vi "Control Documentation.vi"() -> ()   [LabVIEW 2012]
uses:
  Control Documentation.ctl
  <vilib>/regexp/Match Regular Expression.xnode
panel:
  out "error out":errorcluster
  out "Progress":i32(slide) scale=0.0..64.0
  in  "Ignore":bool
  in  "Write":bool
  in  "File Folder":path=path "C:/Users/husmith/Documents/GitHub/iWorx/LabVIEW"
  out "Found Controls":T1(array[cluster])
  in  "Control Documentation":T2[](array[typedef])=[{"Label"="Channel", "Tip Strip"="Select the iWorx sensor adaptor channel", "Description"="Select the channel for the iWorx sensor adaptor. Chanel 1 is read on AI0 channel 2 is read on AI1."}, {"Label"="Raw Signal", "Tip Strip"="The raw voltage signal from the sensor", "Description"="This control shows the raw voltage signal from the myDAQ before any scaling is applied."}, {"Label"="Sample Timing", "Tip Strip"="Select how frequently to read data", "Description"="Set the approximate read frequency for the data acquisition functions."}, {"Label"="Set Up", "Tip Strip"="Open sensor set up instructions", "Description"=""}, {"Label"="Calibration Data", "Tip Strip"="Calibration set points", "Description"="The set points are used to calulate a linear slope and offset using the formulas below.\nSlope = (X2-X1)/(Y2-Y1)\nOffset = (X1-(slope*Y1)\nScaled Data = Data*m+b"}, {"Label"="Set SP1", "Tip Strip"="Save current raw voltage as set point 1 voltage", "Description"=""}, {"Label"="Set SP2", "Tip Strip"="Save current raw voltage as set point 1 voltage", "Description"=""}, {"Label"="Slope", "Tip Strip"="The slope calculated using the calibration data", "Description"=""}, {"Label"="Offset", "Tip Strip"="The offset calculated using the calibration data", "Description"=""}, {"Label"="Autoscale Y", "Tip Strip"="Toggle Y axis autoscaling", "Description"=""}, {"Label"="Open Log", "Tip Strip"="Open the current chart data in Excel", "Description"="Note: This feature will not work if Microsoft Excel is not installed."}, {"Label"="Clear Chart", "Tip Strip"="Clear the waveform chart data", "Description"=""}, {"Label"="Processed Signal", "Tip Strip"="The scaled sensor data", "Description"=""}, {"Label"="Waveform Chart", "Tip Strip"="", "Description"=""}, {"Label"="Snapshot", "Tip Strip"="Take a snapshot of the graph and save to file", "Description"=""}, {"Label"="Pause Button", "Tip Strip"="Pause the waveform chart", "Description"=""}, {"Label"="stop", "Tip Strip"="Stop the VI", "Description"=""}]
  out "All Controls":string[](array[string])
  out "File Path Control":path=path "C:/Users/husmith/Documents/GitHub/iWorx/LabVIEW/examples/iWorx - Force.vi"
  in  "Background":bool
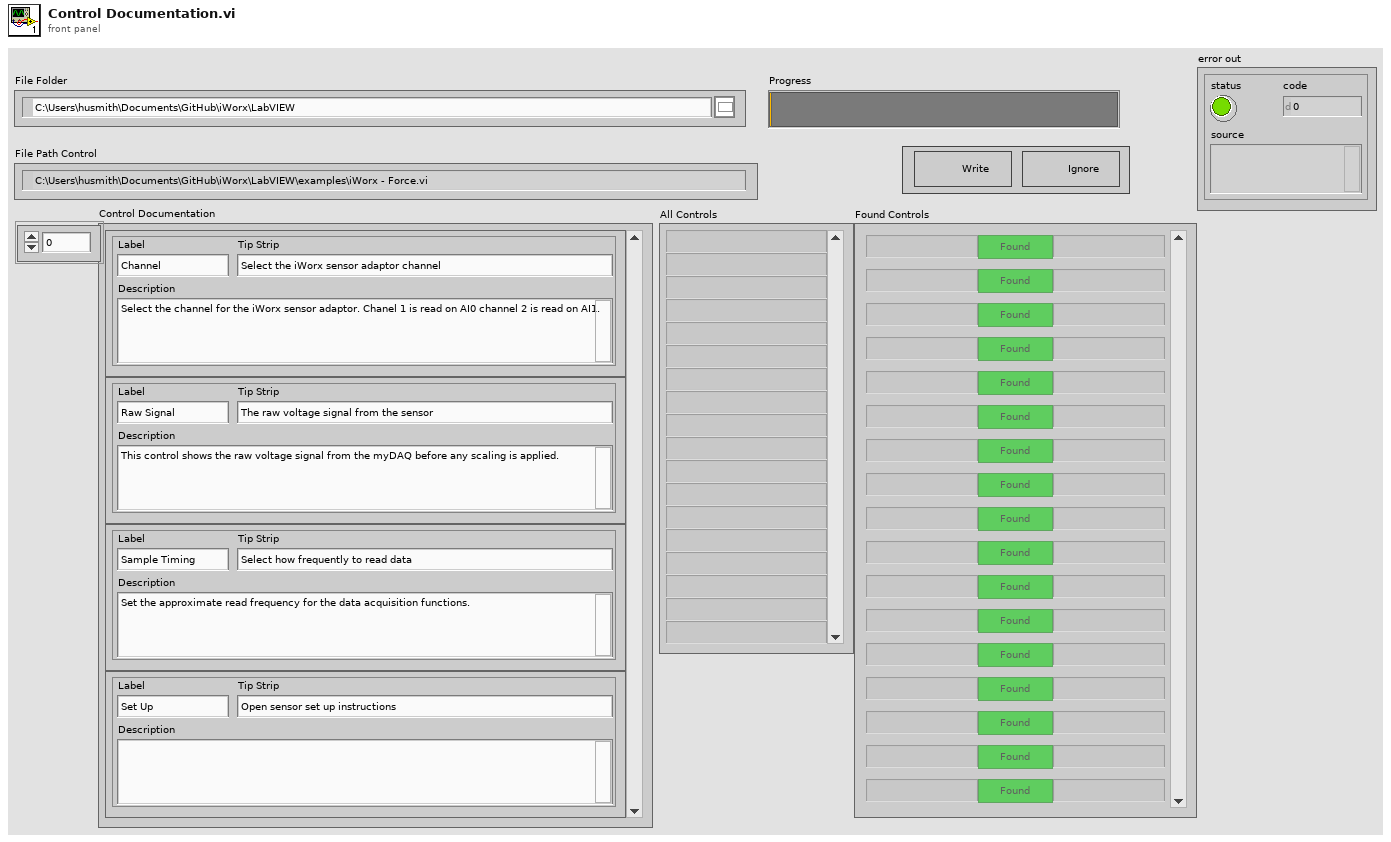
[diagram p1: front panel]
types:
  T1 = cluster{"Label":string, "Found":bool, "Found Label":string}[]
  T2 = typedef "Control Documentation.ctl" = cluster{"Label":string, "Tip Strip":string, "Description":string}
  T3 = cluster{"Label":string, "Found":bool, "Found Label":string}
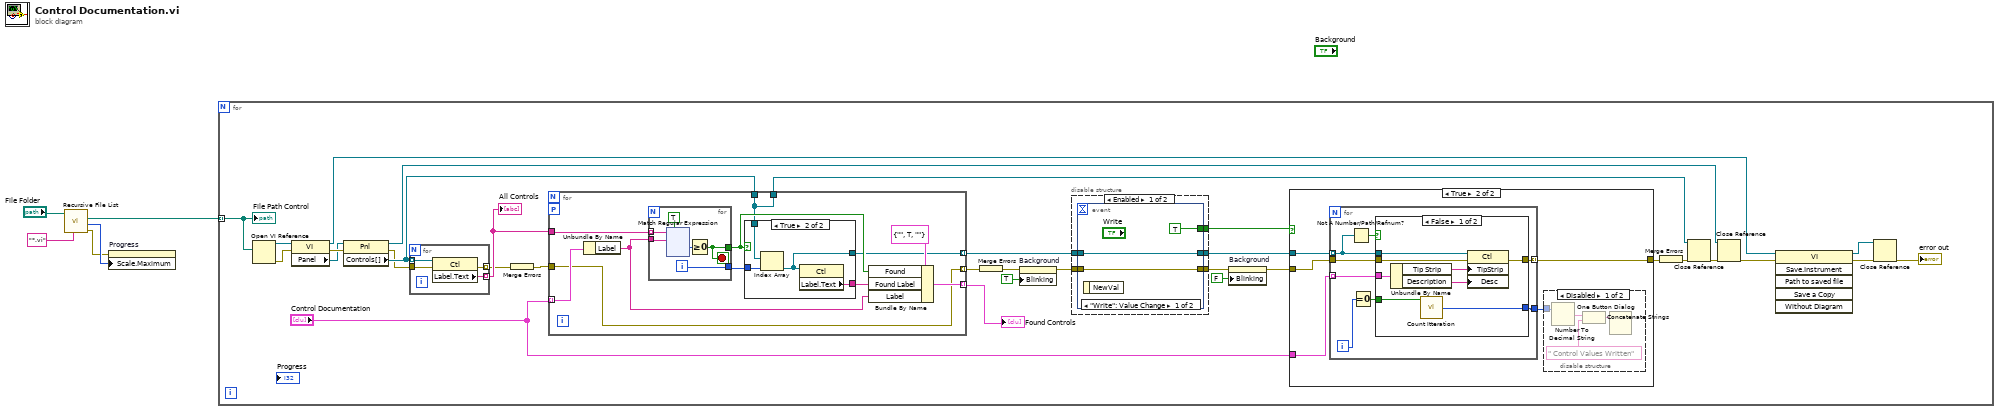
[diagram p0: block diagram]
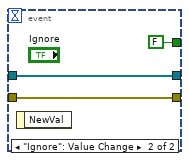
[diagram p2: hidden frame]
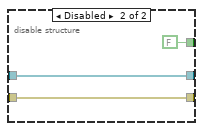
[diagram p3: hidden frame]
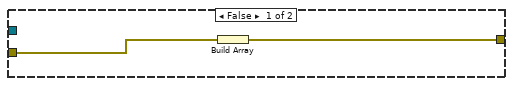
[diagram p4: hidden frame]
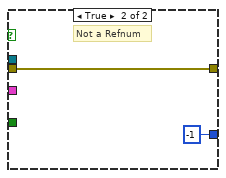
[diagram p6: hidden frame]
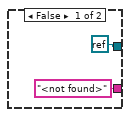
[diagram p7: hidden frame]
diagram:
  n1 = call <vilib>:"Recursive File List.vi"("pattern"="*.vi", "Folder Path"="File Folder") -> ("error out"=w2:errorcluster, "Number of Files"=w3:i32, "All Files in Dir"=w1:path[])  [unwired: 5 in, 2 out]
  n2 = property on="Progress" class="Slide (strict)"(error in=w2, "Scale.Maximum"=w3) -> ()  [unwired: 1 in, 2 out]
  n3 = for {
    tunnel: w1 -> [w10] mode=indexing
    n4 = Open VI Reference(vi path=w10) -> (vi reference=w33:refnum<vi>, error out=w37:errorcluster)  [unwired: 5 in]
    n5 = property on="Property Node" class="VI"(reference=w33, error in=w37) -> (reference out=w8:refnum<vi>, error out=w36:errorcluster, "Panel"=w35:refnum<vi>)
    n6 = property on="Property Node" class="Pnl"(reference=w35, error in=w36) -> (reference out=w32:refnum<vi>, error out=w27:errorcluster, "Controls[]"=w30:refnum<vi>[])
    n7 = for {
      tunnel: w30 -> [w218] mode=indexing
      tunnel: [w217] -> w34 mode=indexing
      tunnel: w27 -> [w216]
      tunnel: [w215] -> w21 mode=indexing
      n8 = property on="Property Node" class="Ctl"(reference=w218, error in=w216) -> (error out=w215:errorcluster, "Label.Text"=w217:string)  [unwired: 1 out]
    }
    "All Controls" <- w34
    n9 = Merge Errors(w21) -> (w20:errorcluster)
    n10 = for {
      tunnel: w34 -> [w91]
      tunnel: "Control Documentation" -> [w90] mode=indexing
      tunnel: w30 -> [w83]
      tunnel: [w85] -> w29 mode=indexing
      tunnel: [w83] -> w28
      tunnel: [w82] -> w25 mode=indexing
      tunnel: w20 -> [w81]
      tunnel: [w81] -> w19 mode=indexing
      workers-P: _ -> [_]
      n11 = Unbundle By Name(w90) -> ("Label"=w84:string)
      n12 = for {
        tunnel: w91 -> [w103] mode=indexing
        tunnel: [w102] -> w89
        tunnel: w84 -> [w101]
        tunnel: [w99] -> w87
        i -> [w102]
        stop <- w99 stop-if-true
        n13 = xnode "Match Regular Expression"("input string"=w103, "regular expression"=w101, "ignore case? (F)"=TRUE) -> ("offset past match"=w100:i32)  [unwired: 3 in, 4 out]
        n14 = Greater Or Equal To 0?(x=w100) -> (x >= 0?=w99:bool)
      }
      n15 = case shown="True" w87 {
        tunnel: w83 -> [_ w97]
        tunnel: w89 -> [_ w96]
        tunnel: ["<not found>" ("Label.Text") w95] -> w86
        tunnel: [refnum<k0> refnum w94] -> w82
        frame False {
        }
        frame True {
          n16 = Index Array(array=w97, index=w96) -> (element=w94:refnum<vi>)
          n17 = property on="Property Node" class="Ctl"(reference=w94) -> ("Label.Text"=w95:string)  [unwired: 1 in, 2 out]
        }
      }
      n18 = Bundle By Name(cluster=T3 {"Label"="", "Found"=TRUE, "Found Label"=""} ("Controls"), "Found"=w87, "Found Label"=w86, "Label"=w84) -> (w85:T3)
    }
    "Found Controls" <- w29
    n19 = Merge Errors(w19) -> (w18:errorcluster)
    n20 = property on="Background" class="Bool"(error in=w18, "Blinking"=TRUE) -> (error out=w17:errorcluster)  [unwired: 1 in, 1 out]
    n21 = disable-structure shown="Enabled" {
      disable-tunnel: w25 -> [w42 w51]
      disable-tunnel: [w41 FALSE] -> w24
      disable-tunnel: [w40 w51] -> w23
      disable-tunnel: w17 -> [w39 w50]
      disable-tunnel: [w38 w50] -> w15
      frame Enabled {
        n22 = event shown="[0] \"Write\": Value Change" {
          selector: _ -> [_ _]
          dyn-events: _ -> [_ _]
          timeout: _ -> [_ _]
          tunnel: w42 -> [w44 w47]
          tunnel: [TRUE FALSE] -> w41
          tunnel: [w44 w47] -> w40
          tunnel: w39 -> [w43 w46]
          tunnel: [w43 w46] -> w38
          event "Write": Value Change {
            n23 = event-data() -> ()  [unwired: 1 in, 1 out]
          }
          event "Ignore": Value Change {
            n24 = event-data() -> ()  [unwired: 1 in, 1 out]
          }
        }
      }
      frame Disabled {
      }
    }
    n25 = property on="Background" class="Bool"(error in=w15, "Blinking"=FALSE) -> (error out=w14:errorcluster)  [unwired: 1 in, 1 out]
    n26 = case shown="True" w24 {
      tunnel: "Control Documentation" -> [_ w58]
      tunnel: w23 -> [_ w57]
      tunnel: w14 -> [w53 w55]
      tunnel: [w52 w56] -> w13
      frame False {
        n27 = Build Array(w53) -> (w52:errorcluster[])
      }
      frame True {
        n28 = for {
          tunnel: w57 -> [w70] mode=indexing
          tunnel: w58 -> [w68] mode=indexing
          tunnel: [w67] -> w56 mode=indexing
          tunnel: w55 -> [w66]
          tunnel: [w65] -> w54
          i -> [w64]
          n29 = Not A Number/Path/Refnum?(number/path/refnum=w70) -> (NaN/Path/Refnum?=w69:bool)
          n30 = Equal To 0?(x=w64) -> (x = 0?=w63:bool)
          n31 = case shown="False" w69 {
            tunnel: w70 -> [w78 _]
            tunnel: w68 -> [w77 _]
            tunnel: [w74 w80] -> w67
            tunnel: w66 -> [w73 w80]
            tunnel: [w72 -1 ("Itteration")] -> w65
            tunnel: w63 -> [w71 _]
            frame False {
              n32 = Unbundle By Name(w77) -> ("Tip Strip"=w75:string, "Description"=w76:string)
              n33 = call <userlib>:"Count Itteration.vi"("Reset"=w71) -> ("Itteration"=w72:i32)  [unwired: 6 in, 1 out]
              n34 = property on="Property Node" class="Ctl"(reference=w78, error in=w73, "TipStrip"=w75, "Desc"=w76) -> (error out=w74:errorcluster)  [unwired: 1 out]
            }
            frame True {
              # "Not a Refnum"
            }
          }
        }
        n35 = disable-structure shown="Disabled" {
          disable-tunnel: w54 -> [w60 _]
          frame Disabled {
            n36 = Number To Decimal String(number=w60) -> (decimal integer string=w59:string)  [unwired: 1 in]
            n37 = Concatenate Strings(w59, " Control Values Written" ("message")) -> (w61:string)
            n38 = One Button Dialog(message=w61) -> ()  [unwired: 1 in, 1 out]
          }
          frame Enabled {
          }
        }
      }
    }
    n39 = Merge Errors(w13) -> (w12:errorcluster)
    n40 = Close Reference(reference=w28, error in (no error)=w12) -> (error out=w31:errorcluster)
    n41 = Close Reference(reference=w32, error in (no error)=w31) -> (error out=w9:errorcluster)
    n42 = invoke class="VI" method="Save.Instrument"(reference=w8, error in=w9) -> (reference out=w6:refnum<vi>, error out=w7:errorcluster)  [unwired: 4 in, 4 out]
    n43 = Close Reference(reference=w6, error in (no error)=w7) -> (error out=→"error out":errorcluster)
    "File Path Control" <- w10
  }
